vi "set units.vi"(5 "Current Rule":i32(listbox), 6 "Current State":i32(listbox), 7 "Rules":T1=[{"state rules"=[{"next state"=0, "conditions"=[], "number of conditions"=0, "Rule name"=""}, {"next state"=1, "conditions"=[{"> or <"=FALSE, "set point"=500, "sensors and variables"=0, "Data average interval"=0.0}], "number of conditions"=1, "Rule name"=""}, {"next state"=1, "conditions"=[{"> or <"=FALSE, "set point"=10, "sensors and variables"=0, "Data average interval"=0.0}, {"> or <"=FALSE, "set point"=10, "sensors and variables"=0, "Data average interval"=0.0}, {"> or <"=TRUE, "set point"=20, "sensors and variables"=0, "Data average interval"=0.0}, {"> or <"=TRUE, "set point"=500, "sensors and variables"=0, "Data average interval"=0.0}], "number of conditions"=4, "Rule name"=""}], "State name"=""}, {"state rules"=[{"next state"=1, "conditions"=[{"> or <"=FALSE, "set point"=0, "sensors and variables"=0, "Data average interval"=0.0}], "number of conditions"=1, "Rule name"=""}, {"next state"=0, "conditions"=[{"> or <"=FALSE, "set point"=0, "sensors and variables"=0, "Data average interval"=0.0}], "number of conditions"=4, "Rule name"=""}], "State name"=""}] {"state rules"."number of conditions" min=1 step=1; "state rules"."conditions"."Data average interval" min=0.0 format="%^#_3g"; "state rules"."conditions"."sensors and variables" items=["Elapsed time in current state"]; "state rules"."next state" items=["john", "dick"]}) -> (0 "State names":string[](array[string]), 1 "Rule names":string[](array[string]), 2 "number of conditions":u8, 3 "Rules out":T1=[{"state rules"=[{"next state"=0, "conditions"=[], "number of conditions"=0, "Rule name"=""}, {"next state"=1, "conditions"=[{"> or <"=FALSE, "set point"=500, "sensors and variables"=0, "Data average interval"=0.0}], "number of conditions"=1, "Rule name"=""}, {"next state"=1, "conditions"=[{"> or <"=FALSE, "set point"=10, "sensors and variables"=0, "Data average interval"=0.0}, {"> or <"=FALSE, "set point"=10, "sensors and variables"=0, "Data average interval"=0.0}, {"> or <"=TRUE, "set point"=20, "sensors and variables"=0, "Data average interval"=0.0}, {"> or <"=TRUE, "set point"=500, "sensors and variables"=0, "Data average interval"=0.0}], "number of conditions"=4, "Rule name"=""}], "State name"=""}, {"state rules"=[{"next state"=1, "conditions"=[{"> or <"=FALSE, "set point"=0, "sensors and variables"=0, "Data average interval"=0.0}], "number of conditions"=1, "Rule name"=""}, {"next state"=0, "conditions"=[{"> or <"=FALSE, "set point"=0, "sensors and variables"=0, "Data average interval"=0.0}], "number of conditions"=4, "Rule name"=""}], "State name"=""}] {"state rules"."number of conditions" min=1 step=1; "state rules"."conditions"."Data average interval" min=0.0 format="%^#_3g"; "state rules"."conditions"."sensors and variables" items=["Elapsed time in current state"]; "state rules"."next state" items=["john", "dick"]})   [LabVIEW 2019]
uses:
  rules.ctl
  State rules.ctl
  rule.ctl
  condition.ctl
  greater or less.ctl
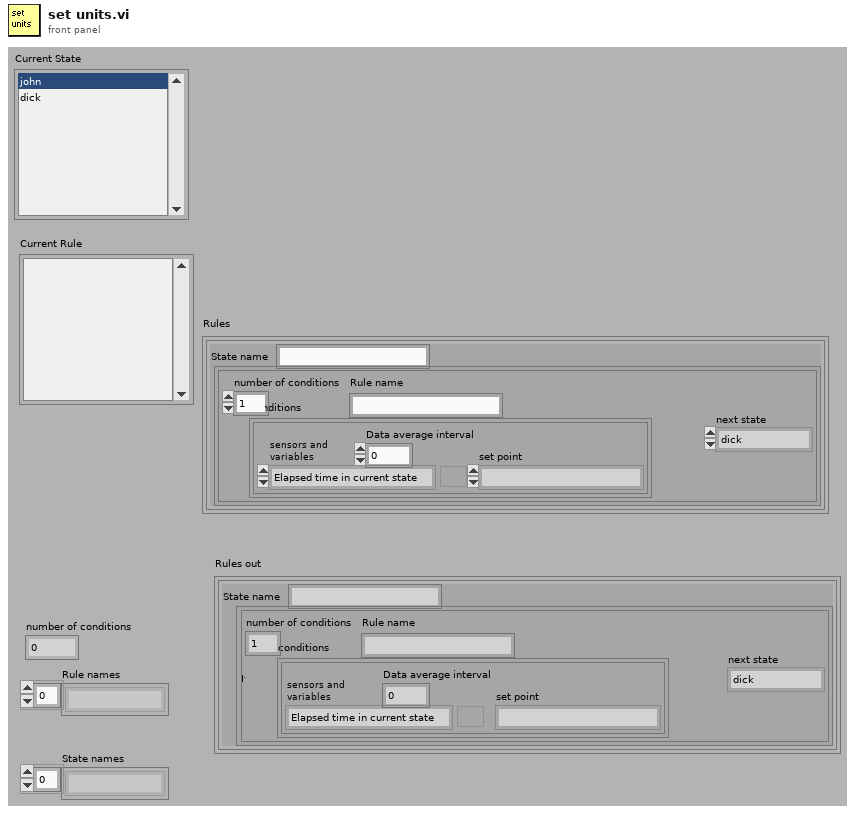
[diagram p1: front panel]
types:
  T1 = typedef "rules.ctl" = T2[]
  T2 = typedef "State rules.ctl" = cluster{"state rules":T3[], "State name":string}
  T3 = typedef "rule.ctl" = cluster{"next state":u16, "conditions":T4[], "number of conditions":u8, "Rule name":string}
  T4 = typedef "condition.ctl" = cluster{"> or <":T5, "set point":i32, "sensors and variables":i32, "Data average interval":dbl}
  T5 = typedef "greater or less.ctl" = bool
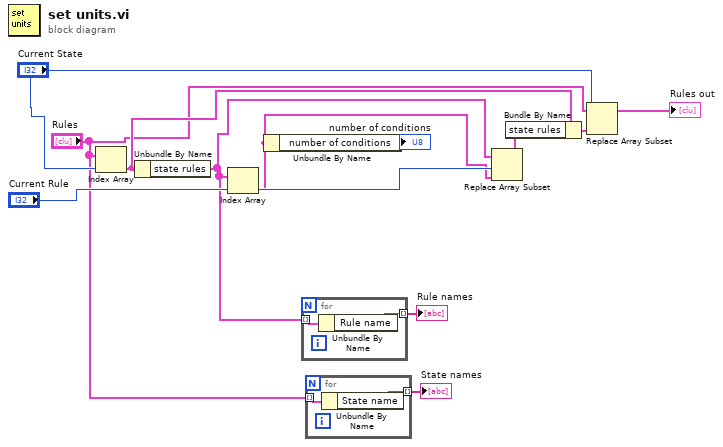
[diagram p0: block diagram]
diagram:
  n1 = Index Array(array="Rules", index="Current State") -> (element=w7:T2)
  n2 = Unbundle By Name(w7) -> ("state rules"=w6:T3[])
  n3 = Index Array(array=w6, index="Current Rule") -> (element=w1:T3)
  n4 = Unbundle By Name(w1) -> ("number of conditions"=→"number of conditions":u8)
  n5 = for {
    tunnel: w6 -> [w14] mode=indexing
    tunnel: [w13] -> w5 mode=indexing
    n6 = Unbundle By Name(w14) -> ("Rule name"=w13:string)
  }
  "Rule names" <- w5
  n7 = for {
    tunnel: "Rules" -> [w16] mode=indexing
    tunnel: [w15] -> w2 mode=indexing
    n8 = Unbundle By Name(w16) -> ("State name"=w15:string)
  }
  "State names" <- w2
  n9 = Replace Array Subset(array=w6, new element=w1, index="Current Rule") -> (w11:T3[])
  n10 = Bundle By Name(cluster=w7, "state rules"=w11) -> (w10:T2)
  n11 = Replace Array Subset(array="Rules", new element=w10, index="Current State") -> (→"Rules out":T1)
